vi "WebPage Addon.Async.vi"(10 "Parameters":variant, 11 "Process":refnum<class "Process.lvclass">) -> ()   [LabVIEW 2026, in "WebPage Addon Engine.lvlib"]
uses:
  WebPage Addon Engine.lvlib
  <vilib>/NI/NIVS Inline Async API/_VS Inline Async API/Process/Process.lvclass
  Addon Shared/Types/Compiled.Settings.ctl
  <vilib>/NI/NIVS Inline Async API/_VS Inline Async API/Process/Process.lvclass/Process.ctl
  <vilib>/NI/NIVS Inline Async API/_Data Access Engine/Access Type Classes/Read/Read.lvclass/Read.ctl
  <vilib>/NI/NIVS Inline Async API/_Data Access Engine/Data Access Engine/Methods/Read.Data.vi
  <vilib>/NI/NIVS Inline Async API/_VS Inline Async API/Process/Data Member Access/Read Data Access.vi
  <vilib>/NI/NIVS Inline Async API/_VS Inline Async API/Error Handling Process/SubVIs/Error.ConvertArray.vi
  <vilib>/NI/NIVS Inline Async API/_Data Access Engine/Access Type Classes/Read/Read.ProcessData.vi
  <vilib>/Utility/error.llb/Trim Whitespace.vi
  <vilib>/Utility/error.llb/Trim Whitespace (string).vi
  <vilib>/Utility/error.llb/Trim Whitespace One-Sided.vi
  Addon Shared/Constants.vi
  <vilib>/Utility/SystemLogging/Write to System Log.vi
  <vilib>/NI/NIVS Inline Async API/_Data Access Engine/Data Access Engine/Methods/Read.Lookup.vi
  gRPCWebPageInterface.lvlibp/Client API/Create Client.vi
  gRPCWebPageInterface.lvlibp/RPC Service/DashboardControl/DashboardControl Shutdown.vi
  gRPCWebPageInterface.lvlibp/Client API/Destroy Client.vi
  <vilib>/NI/NIVS Inline Async API/_Data Access Engine/Data Access Engine/Data Access Engine.lvclass
  Addon Shared/WebPage Addon Shared.lvlib
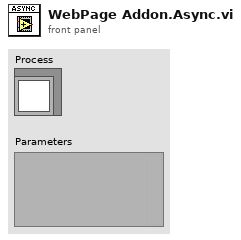
[diagram p1: front panel]
types:
  T1 = typedef "WebPage Addon Shared.lvlib/Compiled.Settings.ctl" = cluster{"Name":string, "Decimation":u32, "Channel Names":string[], "Hosted IP Address":string, "Hosted Port":u32, "gRPC Port":u32}
  T2 = typedef "Data Access Engine.lvlib/Data Access Engine.lvclass/Read.DVR.ctl" = refnum<data-value>
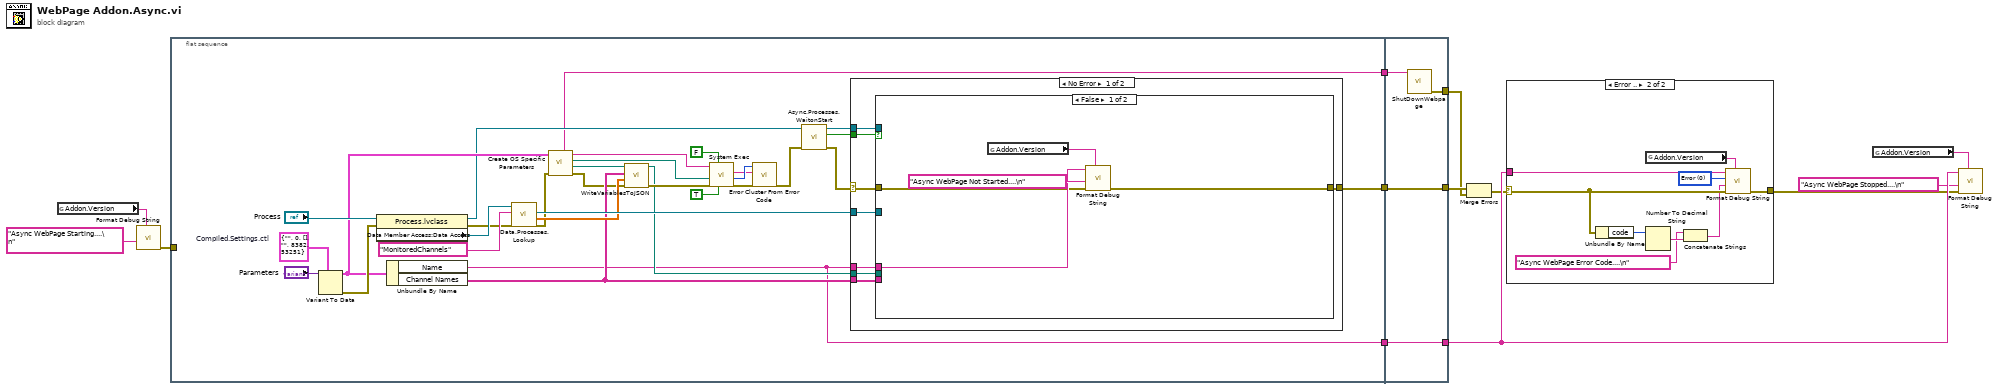
[diagram p0: block diagram]
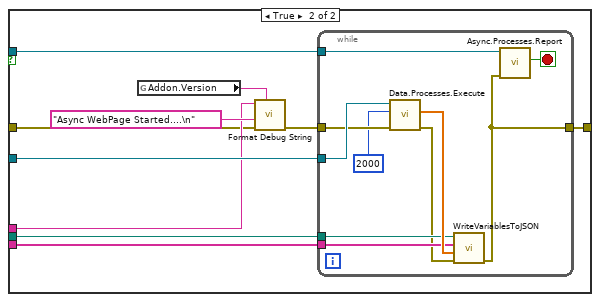
[diagram p2: hidden frame]
diagram:
  n1 = global read "Constants.vi" "Addon.Version"() -> (w9:string)
  n2 = call "Format Debug String.vi"("Version"=w9, "State"="Async WebPage Starting....\n") -> ("error out"=w7:errorcluster)  [unwired: 9 in]
  n3 = flat-sequence {
    tunnel: [w14] -> w13
    tunnel: [w20] -> w12
    tunnel: w7 -> [_]
    tunnel: [w19] -> w5
    tunnel: [w82] -> w10
    tunnel: w13 -> [w81]
    tunnel: w12 -> [w80]
    tunnel: [w80] -> w11
    tunnel: [w79] -> w6
    tunnel: w5 -> [w79]
    frame #0 {
      w37 = T1 {"Name"="", "Decimation"=0, "Channel Names"=[], "Hosted IP Address"="", "Hosted Port"=8382, "gRPC Port"=53251}  # Compiled.Settings.ctl
      n4 = Variant To Data(type=w37, Variant="Parameters") -> (data=w24:T1, error out=w36:errorcluster)  [unwired: 1 in]
      n5 = property class="Process.lvclass"(reference="Process", error in=w36) -> (reference out=w18:refnum<class "Process.lvclass">, error out=w30:errorcluster, "Data Member Access:Data Access"=w39:refnum<class "Data Access Engine.lvclass">)
      n6 = Unbundle By Name(w24) -> ("Name"=w19:string, "Channel Names"=w27:string[])
      n7 = call-poly <vilib>:"Data.Processes.Lookup.vi"("error in (no error)"=w30, "Name"="MonitoredChannels", "Data Access API in"=w39) -> ("error out"=w23:errorcluster, "Initial Values"=w29:dbl[], "Ref"=w41:T2)  [unwired: 5 in, 1 out]
      n8 = call "Create OS Specific Parameters.vi"("error in (no error)"=w23, "Compiled.Settings"=w24) -> ("error out"=w22:errorcluster, "json path"=w17:path, "webpage directory"=w15:path, "start cmd"=w16:string, "gRPC address"=w14:string)  [unwired: 5 in]
      n9 = call "WriteVariablesToJSON.vi"("error in"=w22, "Channel Values"=w29, "Channel Names"=w27, "path"=w17) -> ("error out"=w31:errorcluster, "path out"=w26:path)  [unwired: 6 in]
      n10 = call <vilib>:"System Exec.vi"("run minimized? (F)"=TRUE, "wait until completion? (T)"=FALSE, "error in (no error)"=w31, "working directory"=w15, "command line"=w16) -> ("error out"=w32:errorcluster, "return code"=w33:i32, "standard error"=w21:string)  [unwired: 3 in, 1 out]
      n11 = call <vilib>:"Error Cluster From Error Code.vi"("error in (no error)"=w32, "error message (\"\")"=w21, "error code (0)"=w33) -> ("error out"=w28:errorcluster)  [unwired: 6 in]
      n12 = call <vilib>:"Async.Processes.WaitonStart.vi"("error in (no error)"=w28, "Process"=w18) -> ("error out"=w42:errorcluster, "Execute"=w44:bool, "Process out"=w43:refnum<class "Process.lvclass">)  [unwired: 7 in]
      n13 = case shown="No Error" w42 {
        selector: w42 -> [w46 w78]
        tunnel: w44 -> [w52 _]
        tunnel: w43 -> [w51 _]
        tunnel: w41 -> [w50 _]
        tunnel: w27 -> [w49 _]
        tunnel: w26 -> [w48 _]
        tunnel: [w47 w78] -> w20
        tunnel: w19 -> [w45 _]
        frame No Error {
          n14 = case shown="False" w52 {
            tunnel: w46 -> [w54 w59]
            tunnel: w51 -> [_ w66]
            tunnel: w50 -> [_ w67]
            tunnel: w49 -> [_ w65]
            tunnel: w48 -> [_ w64]
            tunnel: [w53 w63] -> w47
            tunnel: w45 -> [w55 w60]
            frame False {
              n15 = global read "Constants.vi" "Addon.Version"() -> (w57:string)
              n16 = call "Format Debug String.vi"("Version"=w57, "error in (no error)"=w54, "State"="Async WebPage Not Started....\n", "Name"=w55) -> ("error out"=w53:errorcluster)  [unwired: 7 in]
            }
            frame True {
              n17 = global read "Constants.vi" "Addon.Version"() -> (w62:string)
              n18 = call "Format Debug String.vi"("Version"=w62, "error in (no error)"=w59, "State"="Async WebPage Started....\n", "Name"=w60) -> ("error out"=w58:errorcluster)  [unwired: 7 in]
              n19 = while {
                tunnel: w58 -> [w74]
                tunnel: w66 -> [w77]
                tunnel: w67 -> [w75]
                tunnel: w65 -> [w71]
                tunnel: w64 -> [w70]
                tunnel: [w68] -> w63
                stop <- w76 stop-if-true
                n20 = call-poly <vilib>:"Data.Processes.Execute.vi"("error in (no error)"=w74, "timeout ms"=2000, "Ref"=w75) -> ("error out"=w69:errorcluster, "Values"=w72:dbl[])  [unwired: 6 in, 1 out]
                n21 = call "WriteVariablesToJSON.vi"("error in"=w69, "Channel Values"=w72, "Channel Names"=w71, "path"=w70) -> ("error out"=w68:errorcluster)  [unwired: 6 in, 1 out]
                n22 = call <vilib>:"Async.Processes.Report.vi"("Error"=w68, "Process in"=w77) -> ("Stop"=w76:bool)  [unwired: 8 in, 1 out]
              }
            }
          }
        }
        frame Error {
        }
      }
    }
    frame #1 {
      n23 = call "ShutDownWebpage.vi"("address"=w81) -> ("error out"=w82:errorcluster)  [unwired: 9 in, 1 out]
    }
  }
  n24 = Merge Errors(w11, w10) -> (w4:errorcluster)
  n25 = case shown="Error .." w4 {
    selector: w4 -> [w83 w89]
    tunnel: w6 -> [_ w92]
    tunnel: [w83 w84] -> w1
    frame No Error {
    }
    frame Error {
      w90 = 0 items=["Error", "Warning", "Informational"] ("severity (Informational)")
      n26 = Unbundle By Name(w89) -> ("code"=w88:i32)
      n27 = global read "Constants.vi" "Addon.Version"() -> (w91:string)
      n28 = Number To Decimal String(number=w88) -> (decimal integer string=w87:string)  [unwired: 1 in]
      n29 = Concatenate Strings("Async WebPage Error Code....\n" ("State"), w87) -> (w85:string)
      n30 = call "Format Debug String.vi"("Version"=w91, "error in (no error)"=w89, "State"=w85, "severity (Informational)"=w90, "Name"=w92) -> ("error out"=w84:errorcluster)  [unwired: 6 in]
    }
  }
  n31 = global read "Constants.vi" "Addon.Version"() -> (w3:string)
  n32 = call "Format Debug String.vi"("Version"=w3, "error in (no error)"=w1, "State"="Async WebPage Stopped....\n", "Name"=w6) -> ()  [unwired: 7 in, 1 out]
